vi "To JSON Tree.vi"(8 "error in (no error)":errorcluster, 11 "Request in":refnum<class "Request.lvclass">) -> (0 "error out":errorcluster, 2 "JSON out":refnum<class "JSON Null.lvclass">, 3 "Request out":refnum<class "Request.lvclass">)   [LabVIEW 2015, in "Request.lvclass"]
uses:
  Request.lvclass
  <vilib>/NI/JSON Support for LabVIEW/JSON Data Classes/JSON Datatype/JSON Null.lvclass
  Request.lvclass/Request.ctl
  <vilib>/NI/JSON Support for LabVIEW/JSON Data Classes/JSON Object/New JSON Object (Empty).vi
  has params.vi
  <vilib>/NI/JSON Support for LabVIEW/JSON Data Classes/JSON Object/Insert Key Value Pair (Single String).vi
  <vilib>/NI/JSON Support for LabVIEW/JSON Data Classes/JSON Object/Insert Key Value Pair (Single).vi
  id/id.lvclass
  params/params.lvclass
  <vilib>/NI/JSON Support for LabVIEW/JSON Data Classes/JSON Helper/JSON Helper.lvclass
  <vilib>/NI/JSON Support for LabVIEW/JSON Data Classes/JSON Object/JSON Object.lvclass
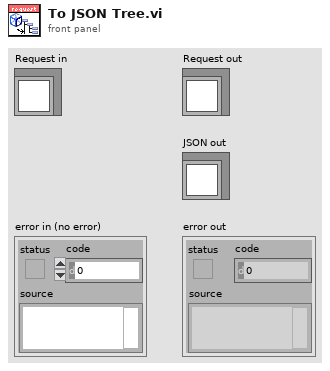
[diagram p1: front panel]
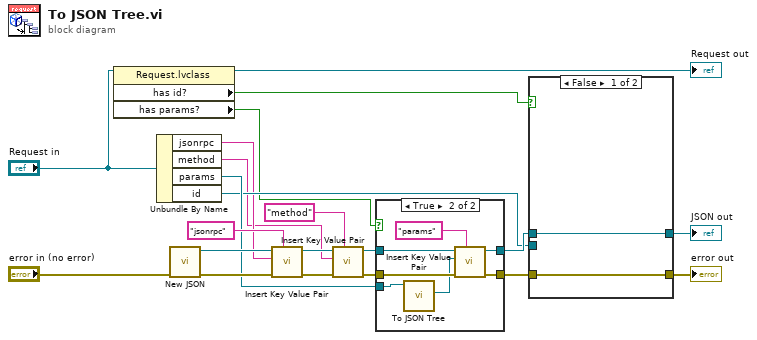
[diagram p0: block diagram]
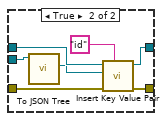
[diagram p2: hidden frame]
diagram:
  n1 = property class="Request.lvclass"(reference="Request in") -> (reference out=→"Request out":refnum<class "Request.lvclass">, "has id?"=w8:bool, "has params?"=w2:bool)  [unwired: 1 in, 1 out]
  n2 = Unbundle By Name("Request in") -> ("jsonrpc"=w7:string, "method"=w6:string, "params"=w10:refnum<class "params.lvclass">, "id"=w9:refnum<class "id.lvclass">)
  n3 = call-poly <vilib>:"New JSON.vi"("error in (no error)"="error in (no error)") -> ("error out"=w13:errorcluster, "JSON Object out"=w14:refnum<class "JSON Object.lvclass">)  [unwired: 9 in]
  n4 = call-poly <vilib>:"Insert Key Value Pair.vi"("key"="jsonrpc", "error in (no error)"=w13, "value"=w7, "JSON Object in"=w14) -> ("error out"=w19:errorcluster, "JSON Object out"=w20:refnum<class "JSON Object.lvclass">)  [unwired: 5 in, 1 out]
  n5 = call-poly <vilib>:"Insert Key Value Pair.vi"("key"="method", "error in (no error)"=w19, "value"=w6, "JSON Object in"=w20) -> ("error out"=w17:errorcluster, "JSON Object out"=w18:refnum<class "JSON Object.lvclass">)  [unwired: 5 in, 1 out]
  n6 = case shown="True" w2 {
    tunnel: w18 -> [w23 w30]
    tunnel: w17 -> [w22 w29]
    tunnel: [w23 w28] -> w16
    tunnel: [w22 w27] -> w15
    tunnel: w10 -> [_ w26]
    frame False {
    }
    frame True {
      n7 = call-dynamic "To JSON Tree.vi"("params in"=w26) -> ("JSON out"=w25:refnum<class "JSON Null.lvclass">)  [unwired: 8 in, 2 out]
      n8 = call-poly <vilib>:"Insert Key Value Pair.vi"("key"="params", "error in (no error)"=w29, "value"=w25, "JSON Object in"=w30) -> ("error out"=w27:errorcluster, "JSON Object out"=w28:refnum<class "JSON Object.lvclass">)  [unwired: 5 in, 1 out]
    }
  }
  n9 = case shown="False" w8 {
    tunnel: w16 -> [w32 w39]
    tunnel: w15 -> [w31 w38]
    tunnel: w9 -> [_ w37]
    tunnel: [w31 w34] -> w4
    tunnel: [w32 w33] -> w3
    frame False {
    }
    frame True {
      n10 = call-dynamic "To JSON Tree.vi"("id in"=w37) -> ("JSON out"=w36:refnum<class "JSON Null.lvclass">)  [unwired: 8 in, 2 out]
      n11 = call-poly <vilib>:"Insert Key Value Pair.vi"("key"="id", "error in (no error)"=w38, "value"=w36, "JSON Object in"=w39) -> ("error out"=w34:errorcluster, "JSON Object out"=w33:refnum<class "JSON Object.lvclass">)  [unwired: 5 in, 1 out]
    }
  }
  "error out" <- w4
  "JSON out" <- w3
